vi "Initialize.vi"(7 "Serial Configuration":T1={"Baud Rate"=9600, "Parity"=0, "Data Bits"=7, "Stop Bits"=10, "Flow Control"=0} {"Flow Control" items=["None", "XON/XOFF", "RTS/CTS", "XON/XOFF & RTS/CTS", "DTR/DSR", "XON/XOFF & DTR/DSR"]; "Stop Bits" items=["1.0"=10, "1.5"=15, "2.0"=20]; "Data Bits" items=["7"=7, "8"=8]; "Parity" items=["None", "Odd", "Even", "Mark", "Space"]; "Baud Rate" items=["300"=300, "600"=600, "1200"=1200, "2400"=2400, "4800"=4800, "9600"=9600, "19200"=19200]}, 8 "error in (no error)":errorcluster, 9 "Reset (True)":bool=TRUE, 10 "ID Query (True)":bool=TRUE, 11 "VISA resource name":refnum<visa-resource-name>) -> (0 "error out":errorcluster, 3 "VISA resource name out":refnum<visa-resource-name>)   [LabVIEW 2019, in "Keithley 6517.lvlib"]
doc: "Establishes communication with the instrument and optionally performs an instrument identification query and/or an instrument reset. It also places the instrument in a default state needed for other instrument driver operations. Therefore, call this VI before calling other instrument driver VIs for this instrument. Generally, you need to call the Initialize VI only once at the beginning of an application."
uses:
  Keithley 6517.lvlib
  Private/Extended User Data.ctl
panel:
  # "(c) 2016-2017 National Instruments.  ALL RIGHTS RESERVED."
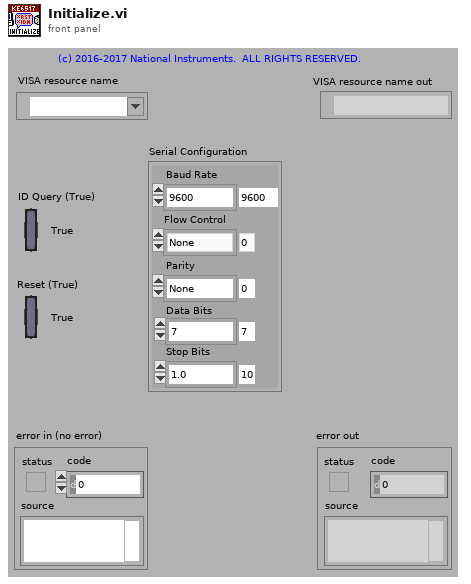
[diagram p1: front panel]
types:
  T1 = cluster{"Baud Rate":u32, "Parity":u16, "Data Bits":u16, "Stop Bits":u16, "Flow Control":u16}
  T2 = typedef "Keithley 6517.lvlib/Extended User Data.ctl" = cluster{"Instrument Model":i32}
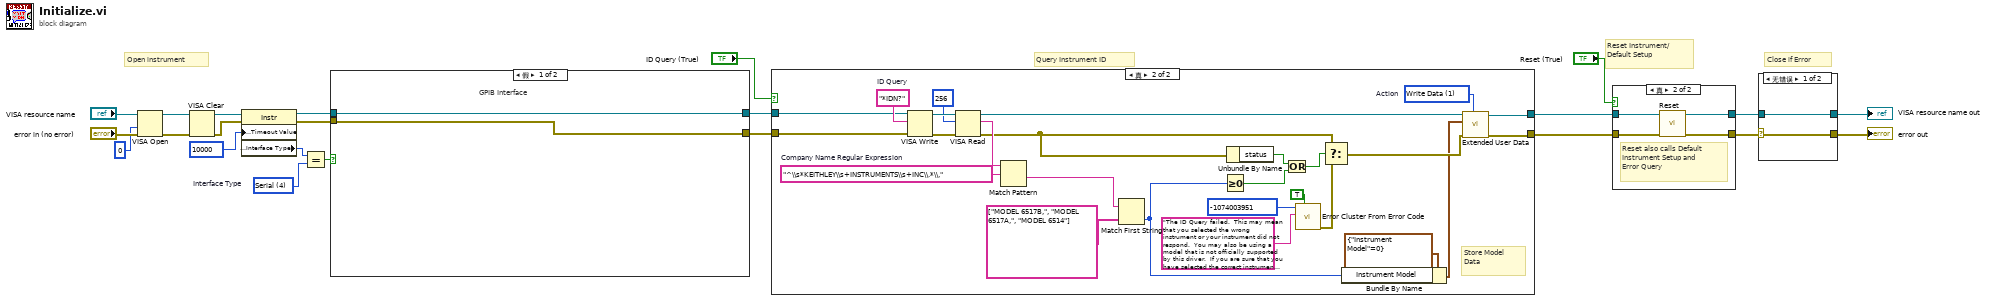
[diagram p0: block diagram]
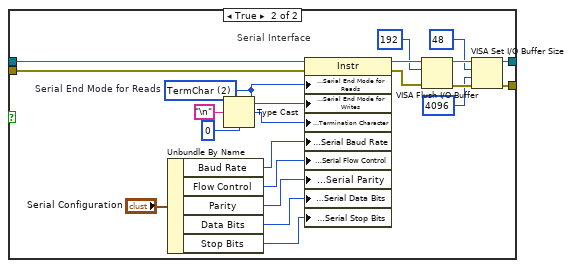
[diagram p2: hidden frame]
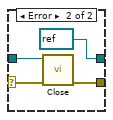
[diagram p3: hidden frame]
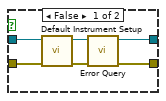
[diagram p4: hidden frame]
diagram:
  w7 = u16 4 items=["GPIB"=1, "VXI"=2, "GPIB-VXI"=3, "Serial"=4, "PXI"=5, "TCPIP"=6, "USB"=7]  # Interface Type
  # "Close if Error"
  # "Query Instrument ID"
  # "Reset Instrument/\nDefault Setup"
  # "Open instrument"
  n1 = VISA Open(access mode=u32 0, error in (no error)="error in (no error)", VISA resource name="VISA resource name") -> (VISA resource name=w18:refnum<visa-resource-name>, error out=w17:errorcluster)  [unwired: 2 in]
  n2 = VISA Clear(VISA resource name=w18, error in (no error)=w17) -> (VISA resource name out=w6:refnum<visa-resource-name>, error out=w5:errorcluster)
  n3 = property class="Instr"(reference=w6, error in=w5, "General Settings:Timeout Value"=u32 10000) -> (reference out=w10:refnum<visa-resource-name>, error out=w9:errorcluster, "Interface Information:Interface Type"=w12:u16)
  n4 = Equal?(x=w12, y=w7) -> (x = y?=w8:bool)
  n5 = case shown="假" w8 {
    tunnel: [w24 w43] -> w4
    tunnel: [w25 w40] -> w3
    tunnel: w10 -> [w24 w45]
    tunnel: w9 -> [w25 w46]
    frame False {
      # "GPIB Interface"
    }
    frame True {
      w33 = u16 2 items=["None", "LastBit", "TermChar"]  # Serial End Mode for Reads
      # "Serial Interface"
      n6 = Unbundle By Name("Serial Configuration") -> ("Baud Rate"=w31:u32, "Flow Control"=w27:u16, "Parity"=w29:u16, "Data Bits"=w30:u16, "Stop Bits"=w26:u16)
      n7 = Type Cast(type=u8 0, x="\n" ("Line Feed Constant")) -> (*(type *) &x=w32:u8)
      n8 = property class="Instr"(reference=w45, error in=w46, "Serial Settings:Serial End Mode for Reads"=w33, "Serial Settings:Serial End Mode for Writes"=w33, "Message Based Settings:Termination Character"=w32, "Serial Settings:Serial Baud Rate"=w31, "Serial Settings:Serial Flow Control"=w27, "Serial Settings:Serial Parity"=w29, "Serial Settings:Serial Data Bits"=w30, "Serial Settings:Serial Stop Bits"=w26) -> (reference out=w39:refnum<visa-resource-name>, error out=w42:errorcluster)
      n9 = VISA Flush I/O Buffer(VISA resource name=w39, mask (16)=u16 192, error in (no error)=w42) -> (VISA resource name out=w44:refnum<visa-resource-name>, error out=w41:errorcluster)
      n10 = VISA Set I/O Buffer Size(VISA resource name=w44, mask (16)=u16 48, size (4096)=u32 4096 ("size (0)"), error in (no error)=w41) -> (VISA resource name out=w43:refnum<visa-resource-name>, error out=w40:errorcluster)
    }
  }
  n11 = case shown="真" "ID Query (True)" {
    tunnel: [w48 w50] -> w2
    tunnel: w4 -> [w48 w58]
    tunnel: w3 -> [w47 w57]
    tunnel: [w47 w51] -> w1
    frame False {
    }
    frame True {
      w54 = u16 1 items=["Read Data", "Write Data", "Clear Data", "Clear ALL Data"]  # Action
      w69 = "*IDN?"  # ID Query
      w71 = "^\\s*KEITHLEY\\s+INSTRUMENTS\\s+INC\\.*\\,"  # Company Name Regular Expression
      # "Store Model\nData"
      n12 = VISA Write(VISA resource name=w58, write buffer=w69, error in (no error)=w57) -> (VISA resource name out=w73:refnum<visa-resource-name>, error out=w72:errorcluster)  [unwired: 1 out]
      n13 = VISA Read(VISA resource name=w73, byte count=u32 256, error in (no error)=w72) -> (VISA resource name out=w53:refnum<visa-resource-name>, read buffer=w74:string, error out=w64:errorcluster)  [unwired: 1 out]
      n14 = Match Pattern(string=w74, regular expression=w71) -> (after substring=w60:string)  [unwired: 1 in, 3 out]
      n15 = Match First String(2:string[] ["MODEL 6517B,", "MODEL 6517A,", "MODEL 6514"] ("string array"), 3:w60) -> (0:w55:i32)  [unwired: 1 out]
      n16 = Greater Or Equal To 0?(x=w55) -> (x >= 0?=w62:bool)
      n17 = Unbundle By Name(w64) -> ("status"=w63:bool)
      n18 = Or(x=w63, y=w62) -> (x .or. y?=w61:bool)
      n19 = call <vilib>:"Error Cluster From Error Code.vi"("show call chain? (False)"=TRUE, "error message (\"\")"="The ID Query failed.  This may mean that you selected the wrong instrument or your instrument did not respond.  You may also be using a model that is not officially supported by this driver.  If you are sure that you have selected the correct instrument and it is responding, try disabling the ID Query." ("Source (VI Name)"), "error code (0)"=-1074003951 ("Code")) -> ("error out"=w68:errorcluster)  [unwired: 6 in]
      n20 = Select(t=w64, s=w61, f=w68) -> (s? t:f=w52:errorcluster)
      n21 = Bundle By Name(cluster=T2 {"Instrument Model"=0} ("User Data Definition"), "Instrument Model"=w55) -> (w49:T2)
      n22 = call "Extended User Data.vi"("Action (0: Read Data)"=w54, "error in (no error)"=w52, "User Data In"=w49, "VISA resource name"=w53) -> ("error out"=w51:errorcluster, "VISA resource name out"=w50:refnum<visa-resource-name>)  [unwired: 5 in, 1 out]
    }
  }
  n23 = case shown="真" "Reset (True)" {
    tunnel: [w78 w84] -> w13
    tunnel: [w79 w83] -> w14
    tunnel: w2 -> [w75 w82]
    tunnel: w1 -> [w76 w81]
    frame False {
      n24 = call "Default Instrument Setup.vi"("error in (no error)"=w76, "VISA resource name"=w75) -> ("error out"=w77:errorcluster, "VISA resource name out"=w80:refnum<visa-resource-name>)  [unwired: 8 in]
      n25 = call "Error Query.vi"("error in (no error)"=w77, "VISA resource name"=w80) -> ("error out"=w78:errorcluster, "VISA resource name out"=w79:refnum<visa-resource-name>)  [unwired: 6 in, 2 out]
    }
    frame True {
      # "Reset also calls Default Instrument Setup and Error Query"
      n26 = call "Reset.vi"("error in (no error)"=w81, "VISA resource name"=w82) -> ("error out"=w84:errorcluster, "VISA resource name out"=w83:refnum<visa-resource-name>)  [unwired: 8 in]
    }
  }
  n27 = case shown="无错误" w13 {
    selector: w13 -> [w85 w88]
    tunnel: w14 -> [w86 w89]
    tunnel: [w86 refnum<visa-resource-name> refnum ("VISA resource name out")] -> w16
    tunnel: [w85 w90] -> w15
    frame No Error {
    }
    frame Error {
      n28 = call "Close.vi"("error in (no error)"=w88, "VISA resource name"=w89) -> ("error out"=w90:errorcluster)  [unwired: 9 in]
    }
  }
  "VISA resource name out" <- w16
  "error out" <- w15
